vi "LuaVIEW Open Private State.vi"(11 "error in (no error)":errorcluster) -> (6 "LuaVIEW reference":T1, 15 "error out":errorcluster)   [LabVIEW 2012]
doc: "Open a LuaVIEW state that does not make use of the public function registry nor any module export functions. To use the returned state, register and set any private and indexed functions, compile a script, and execute it. Once the LuaVIEW reference is no longer required, close it using \"LuaVIEW Close\" to free the associated resources.\n\nThough anything that can be done with a state returned by this function can also be done with a state returned by \"LuaVIEW Open\", it is sometimes desirable to use this VI to prevent the loading of the infrastructure associated with the public function registry.\n\nThe opened LuaVIEW state holds a new instance of the Lua virtual machine. Scripts that run on different LuaVIEW states therefore have separate variable spaces."
uses:
  typedefs/t_LuaVIEW Reference.ctl
  typedefs/et_LuaVIEW CIN Actions.ctl
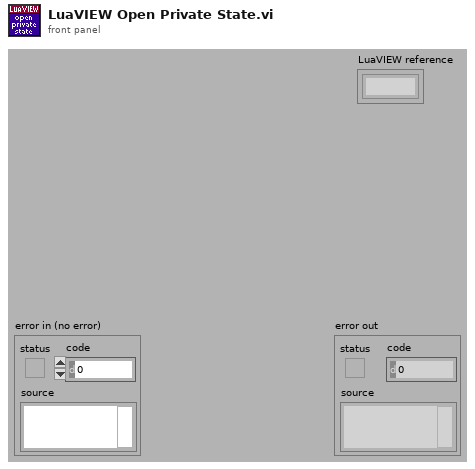
[diagram p1: front panel]
types:
  T1 = typedef "t_LuaVIEW Reference.ctl" = refnum<k1>
  T2 = typedef "et_LuaVIEW CIN Actions.ctl" = enum16{"checksynopsis", "_open", "_registerpublic", "_registerexport", "__never_an_error_result_ns", "luaversion", "cinversion", "_totals", "_taskcount", "pathological", "_unregnextpublic", "registryusecount", "__per_state_actions", "regsetprivate", "regsetindex", "regsetmodule", "_revokeexports", "_usepublic", "prepare", "compile", "execute", "call", "unregstaterefs", "_close", "pullboolean", "pullnumber", "pullI8", "pullU8", "pullI16", "pullU16", "pullI32", "pullU32", "pullobject", "pullrefnum", "pullstring", "pullflat", "pushflat", "pushobject", "getattribute", "setattribute", "stacktostring", "_startyieldtest", "_endyieldtest", "_pollprintbuffer", "__never_an_error_result_ps", "_pollexport", "setclone", "forcecleanup", "gettop", "clearstack", "insert", "pushboolean", "pushnumber", "pushrefnum", "pushstring", "pushnil", "pushvalue", "gettaskref", "settaskref"}
  T3 = typedef "et_LuaVIEW CIN Results.ctl" = enum16{"OK", "error", "main", "call", "clonecall", "modulecall", "exportcall", "index", "yield"}
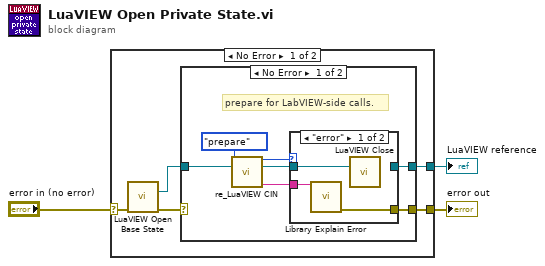
[diagram p0: block diagram]
diagram:
  n1 = case shown="No Error" "error in (no error)" {
    selector: "error in (no error)" -> [w6 w22]
    tunnel: [w8 _] -> w3
    tunnel: [w7 w22] -> w2
    frame No Error {
      n2 = call "LuaVIEW Open Base State.vi"("error in (no error)"=w6) -> ("LuaVIEW reference"=w5:T1, "error out"=w4:errorcluster)  [unwired: 13 in]
      n3 = case shown="No Error" w4 {
        selector: w4 -> [_ w21]
        tunnel: [w11 w20] -> w8
        tunnel: [w10 w21] -> w7
        tunnel: w5 -> [w9 w20]
        frame No Error {
          # "prepare for LabVIEW-side calls."
          n4 = call "re_LuaVIEW CIN.vi"("action"=et_LuaVIEW_CIN_Actions."prepare", "LuaVIEW reference in"=w9) -> ("result"=w14:T3, "LuaVIEW reference out"=w12:T1, "string out"=w13:string)  [unwired: 7 in, 4 out]
          n5 = case shown="\"error\"" w14 {
            tunnel: w13 -> [w17 _]
            tunnel: [w18 _] -> w10
            tunnel: w12 -> [w16 w19]
            tunnel: [_ w19] -> w11
            frame "error" {
              n6 = call "Library Explain Error.vi"("explanation prefix (none)"=w17) -> ("explained error"=w18:errorcluster)  [unwired: 14 in]
              n7 = call "LuaVIEW Close.vi"("LuaVIEW reference"=w16) -> ()  [unwired: 14 in, 1 out]
            }
            frame Default {
            }
          }
        }
        frame Error {
        }
      }
    }
    frame Error {
    }
  }
  "LuaVIEW reference" <- w3
  "error out" <- w2
